vi "test.vi"() -> ()   [LabVIEW 2019]
uses:
  WSCbot_V3_Toolkit.lvlibp/WSCBOTV3_Toolkit/Sensor/LowLevel/IR_Chanel.ctl
  WSCbot_V3_Toolkit.lvlibp
  WSCbot_V3_Toolkit.lvlibp/WSCBOTV3_Toolkit/IO/LowLevel/IO_Chanel_DIO.ctl
  <vilib>/platform/TimedLoop/XDataNode/XDataNode.xnode
  <vilib>/Platform/TimedLoop/XDataNode/nitl_modes.ctl
  <vilib>/Platform/TimedLoop/XDataNode/XDNodeRunTimeDep.lvlib
  <vilib>/Platform/TimedLoop/XDataNode/wakeup.ctl
  <vilib>/Platform/TimedLoop/XDataNode/timing_clust.ctl
panel:
  in  "Stop Button 2":bool
  in  "Stop":bool
  in  "positive/nagative":bool
  in  "Stop Button":bool
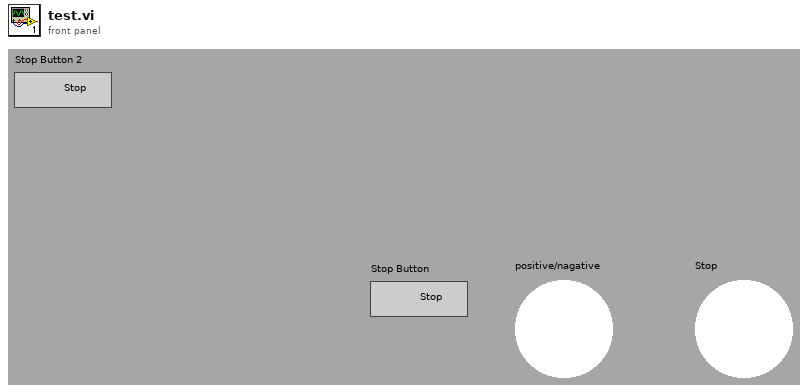
[diagram p1: front panel]
types:
  T1 = typedef "XDNodeRunTimeDep.lvlib/timing_clust.ctl" = cluster{"Expected End [f-1]":u64, "Actual End [f-1]":u64, "Finished Late? [f-1]":bool, "Expected End [i-1]":u64, "Actual End [i-1]":u64, "Finished Late? [i-1]":bool, "Expected Start [i]":u64, "Actual Start [i]":u64, "Expected Start [f]":u64, "Actual Start [f]":u64, "Source Name":string, "Structure Name":string, "Period":i64, "Deadline":i64, "Offset":i64, "Start":i64, "Priority":i32, "Timeout":i32, "Mode":T2, "Wakeup Reason":T3, "Error":errorcluster, "Source Type":string, "Secondary Source Type":string, "Global End Time":u64, "Global Start Time":u64, "Frame Duration":u64, "Iteration Duration":u64, "Assigned CPU":i32, "I/O Scan Engine Mode":u32}
  T2 = typedef "XDNodeRunTimeDep.lvlib/nitl_modes.ctl" = enum32{"No Change", "Process missed periods, maintain original phase", "Discard missed periods, maintain original phase", "Process missed periods, ignore original phase", "Discard missed periods, ignore original phase"}
  T3 = typedef "XDNodeRunTimeDep.lvlib/wakeup.ctl" = enum32{"Normal", "Aborted", "Asynchronous wakeup", "Timing source error", "Timed loop error", "Timeout"}
  T4 = typedef "WSCbot_V3_Toolkit.lvlibp/IO_Chanel_DIO.ctl" = enum16{"A/DIO9", "A/DIO10", "C/DIO0", "C/DIO1", "C/DIO2", "C/DIO3", "C/DIO4", "C/DIO5", "C/DIO6"}
  T5 = typedef "WSCbot_V3_Toolkit.lvlibp/IR_Chanel.ctl" = enum16{"IR_LF", "IR_LB", "IR_BL", "IR_BR", "IR_RB", "IR_RF", "IR_FR", "IR_FL"}
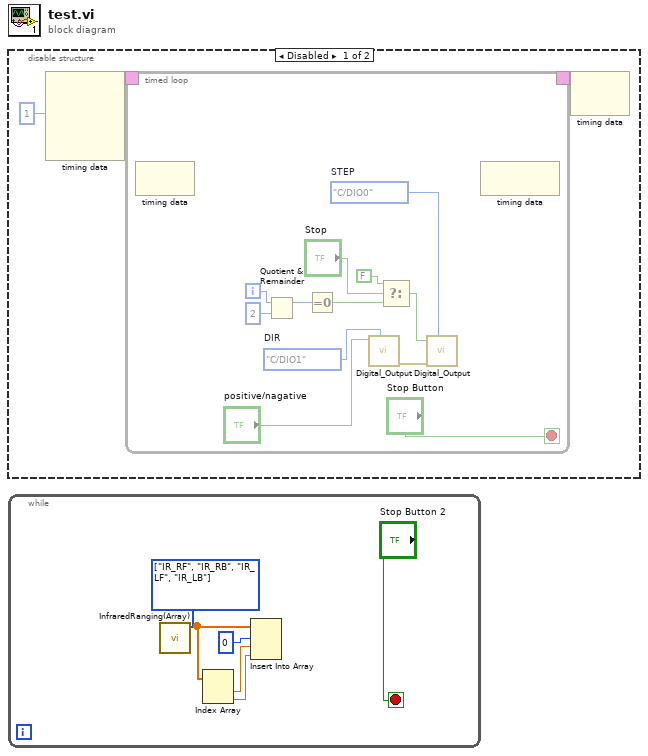
[diagram p0: block diagram]
diagram:
  n1 = disable-structure shown="Disabled" {
    frame Disabled {
      n2 = node-c288(i64 1 ("Period")) -> (w3:T1)  [unwired: 3 in]
      n3 = timed-loop {
        timing: w3 -> [_]
        timing-out: [_] -> w2
        i -> [w7]
        stop <- "Stop Button" stop-if-true
        w14 = IO_Chanel_DIO."C/DIO1"  # DIR
        w15 = IO_Chanel_DIO."C/DIO0"  # STEP
        n4 = node-c288() -> ()  [unwired: 1 in, 1 out]
        n5 = Quotient & Remainder(x=w7, y=2) -> (x-y*floor(x/y)=w5:i32)  [unwired: 1 out]
        n6 = Equal To 0?(x=w5) -> (x = 0?=w4:bool)
        n7 = call "Digital_Output.vi"("IO_Chanel"=w14, "False/True"="positive/nagative") -> ("error out"=w8:errorcluster)  [unwired: 9 in]
        n8 = Select(t=FALSE ("s"), s="Stop", f=w4) -> (s? t:f=w10:bool)
        n9 = call "Digital_Output.vi"("IO_Chanel"=w15, "error in"=w8, "False/True"=w10) -> ()  [unwired: 8 in, 1 out]
        n10 = node-c288() -> ()  [unwired: 1 in, 1 out]
      }
      n11 = node-c288(w2) -> ()  [unwired: 1 out]
    }
    frame Enabled {
    }
  }
  n12 = while {
    stop <- "Stop Button 2" stop-if-true
    w26 = T5[] [enum."IR_RF", enum."IR_RB", enum."IR_LF", enum."IR_LB"] items=["IR_LF", "IR_LB", "IR_BL", "IR_BR", "IR_RB", "IR_RF", "IR_FR", "IR_FL"] ("IR_Chanel")
    n13 = call "InfraredRanging(Array).vi"("IR_Chanel"=w26) -> ("Valtage"=w22:dbl[])  [unwired: 9 in, 1 out]
    n14 = Index Array(array=w22) -> (element #1=w25:dbl, element #2=w24:dbl)  [unwired: 2 in]
    n15 = Insert Into Array(array=w22, index=0, new element #1=w25, new element #2=w24) -> ()  [unwired: 1 out]
  }
